vi "2 midpoint.vi"(9 "UTM 2":T1 {"North" format="%#_10f"; "East" format="%#_8f"}, 11 "UTM 1":T1 {"North" format="%#_10f"; "East" format="%#_8f"}) -> (1 "Distance":dbl, 2 "Midpoint":T1 {"North" format="%#_10f"; "East" format="%#_8f"})   [LabVIEW 2011]
doc: "Returns the midpoint and distance between two UTM locations."
uses:
  2 Typedefs/UTM Location.ctl
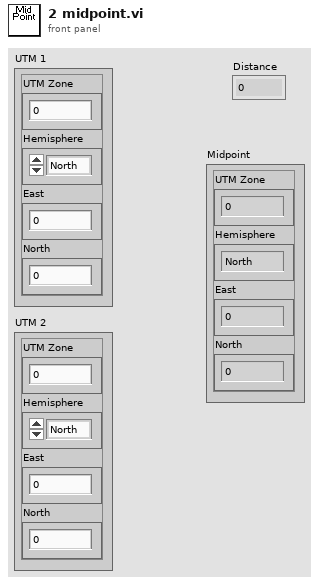
[diagram p1: front panel]
types:
  T1 = typedef "UTM Location.ctl" = cluster{"UTM Zone":dbl, "Hemisphere":enum16{"North", "South"}, "East":dbl, "North":dbl}
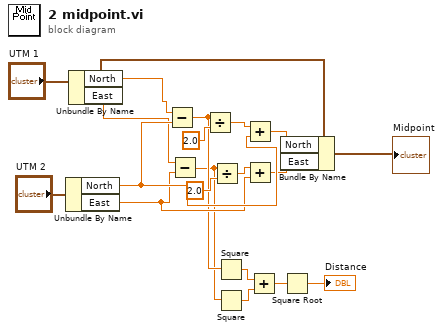
[diagram p0: block diagram]
diagram:
  n1 = Unbundle By Name("UTM 2") -> ("North"=w15:dbl, "East"=w14:dbl)
  n2 = Unbundle By Name("UTM 1") -> ("North"=w11:dbl, "East"=w10:dbl)
  n3 = Subtract(x=w11, y=w15) -> (x-y=w3:dbl)
  n4 = Subtract(x=w10, y=w14) -> (x-y=w2:dbl)
  n5 = Divide(x=w3, y=2.0) -> (x/y=w16:dbl)
  n6 = Divide(x=w2, y=2.0) -> (x/y=w17:dbl)
  n7 = Square(x=w3) -> (x^2=w5:dbl)
  n8 = Square(x=w2) -> (x^2=w6:dbl)
  n9 = Add(x=w16, y=w15) -> (x+y=w12:dbl)
  n10 = Add(x=w17, y=w14) -> (x+y=w13:dbl)
  n11 = Add(x=w5, y=w6) -> (x+y=w4:dbl)
  n12 = Bundle By Name(cluster="UTM 1", "North"=w12, "East"=w13) -> (→"Midpoint":T1)
  n13 = Square Root(x=w4) -> (sqrt(x)=→"Distance":dbl)
